vi "NI 9226 Getting Started (Host).vi"() -> ()   [LabVIEW 2018]
doc: "This VI will initialize the FPGA VI and then continually read and scale to temperature single point values from 4 channels of an analog input module."
uses:
  <vilib>/userdefined/High Color/nirio_resource_hc.ctl
  <vilib>/FPGAPlugInAG/cRIO-9045/niLvFpga_Open_cRIO-9045.vi
  <vilib>/rvi/interface/common/dynamic/niFpgaDynamicAddResources.vi
  <vilib>/FPGAPlugInAG/Dynamic/niLvFpga_Reset_Dynamic.vi
  <vilib>/Utility/error.llb/Error Cluster From Error Code.vi
  <vilib>/rvi/errors/niLvFpgaAdjustHostInterfaceError.vi
  <vilib>/FPGAPlugInAG/Dynamic/niLvFpga_Run_Dynamic.vi
  <vilib>/RVI Host/nirviSupport.llb/nirviErrorClusterFromErrorCode.vi
  <vilib>/FPGAPlugInAG/Dynamic/niLvFpga_Close_Dynamic.vi
  <vilib>/rvi/interface/nirviOpenFPGA/nirviOpenFPGA.xnode
  FPGA Bitfiles/crio_FPGATarget2_NI9226GettingSta_IIeFYHumF2U.lvbitx
  NI 9226 Getting Started (FPGA).vi
  <vilib>/rvi/interface/nirviMethod/nirviMethod.xnode
  <vilib>/rvi/interface/nirviReadWriteControl/nirviReadWriteControl.xnode
  <vilib>/rvi/interface/nirviCloseFPGA/nirviCloseFPGA.xnode
  <vilib>/rvi/interface/Simulation/niFpgaSimulationCallBeginRW.vi
  <vilib>/rvi/interface/nirviMethod/StockFPGA_InlinedMethodWaitForSingleIRQ.vi
  <vilib>/FPGAPlugInAG/Dynamic/niLvFpga_WaitOnIrq_Dynamic.vi
  <vilib>/FPGAPlugInAG/Dynamic/niLvFpga_AcknowledgeIrq_Dynamic.vi
  NiFpgaLv.dll
panel:
  in  "A":dbl=0.003908019978553057 format="%0.5e"
  in  "B":dbl=-5.774199962615967e-07
  in  "C":dbl=-4.182999866625403e-12 format="%0.5e"
  in  "Update":bool
  out "FPGA data transfer timed out":bool
  out "FPGA error out":errorcluster
  out "Host error out":errorcluster
  in  "Conversion Time":enum8{"200 ms", "2.5 ms"}(ring)
  in  "Resource name":T1="RIO0" caption="RIO Device"
  out "Coeff Out of Range":bool
  out "RTD Temperature":T2(graph)
  in  "stop":bool
  # "Overview: This example downloads and runs an FPGA VI that continuously reads single point values from 4 out of the 8 channel of the NI 9226\nRequirements: LabVIEW FPGA Module, LabVIEW Real-Time Module, NI-RIO\nInstructions: \n1) Modify timing parameters if desired . The timming parameters may also be changed during run-time using the \"Update\" button.\n2) Run the VI"
  # "Resource Parameters"
  # "Timing Parameters"
  # "RTD Parameters"
  # "Callendar-Van Dusen Constants"
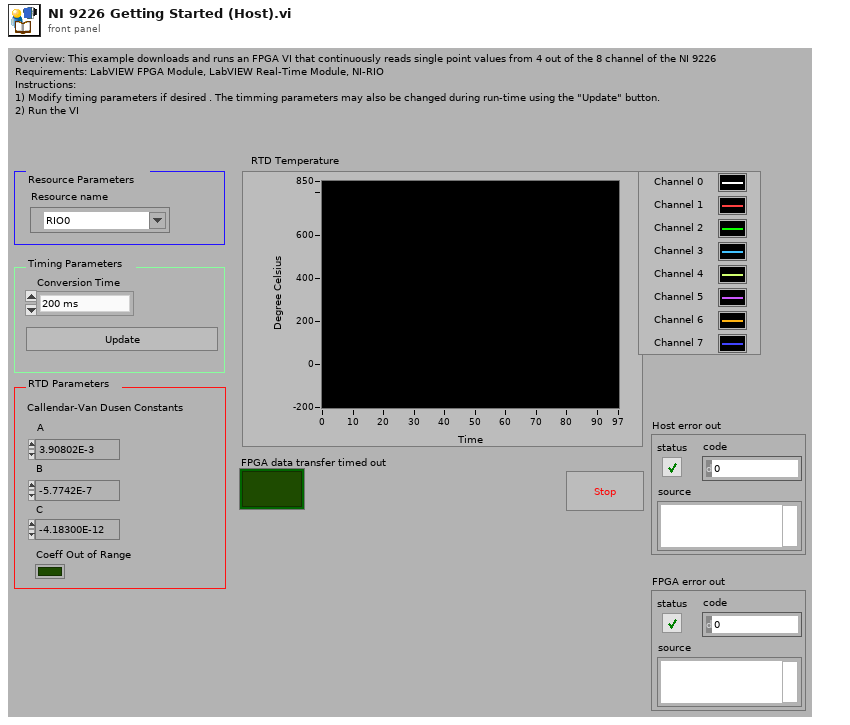
[diagram p1: front panel]
types:
  T1 = typedef "nirio_resource_hc.ctl" = tag
  T2 = cluster{"[0]":dbl, "[1]":dbl, "[2]":dbl, "[3]":dbl}
  T3 = cluster{"Mod6/RTD0":fxp<+/-,24,14>, "Mod6/RTD1":fxp<+/-,24,14>, "Mod6/RTD2":fxp<+/-,24,14>, "Mod6/RTD3":fxp<+/-,24,14>, "Mod6/RTD4":fxp<+/-,24,14>, "Mod6/RTD5":fxp<+/-,24,14>, "Mod6/RTD6":fxp<+/-,24,14>, "Mod6/RTD7":fxp<+/-,24,14>}
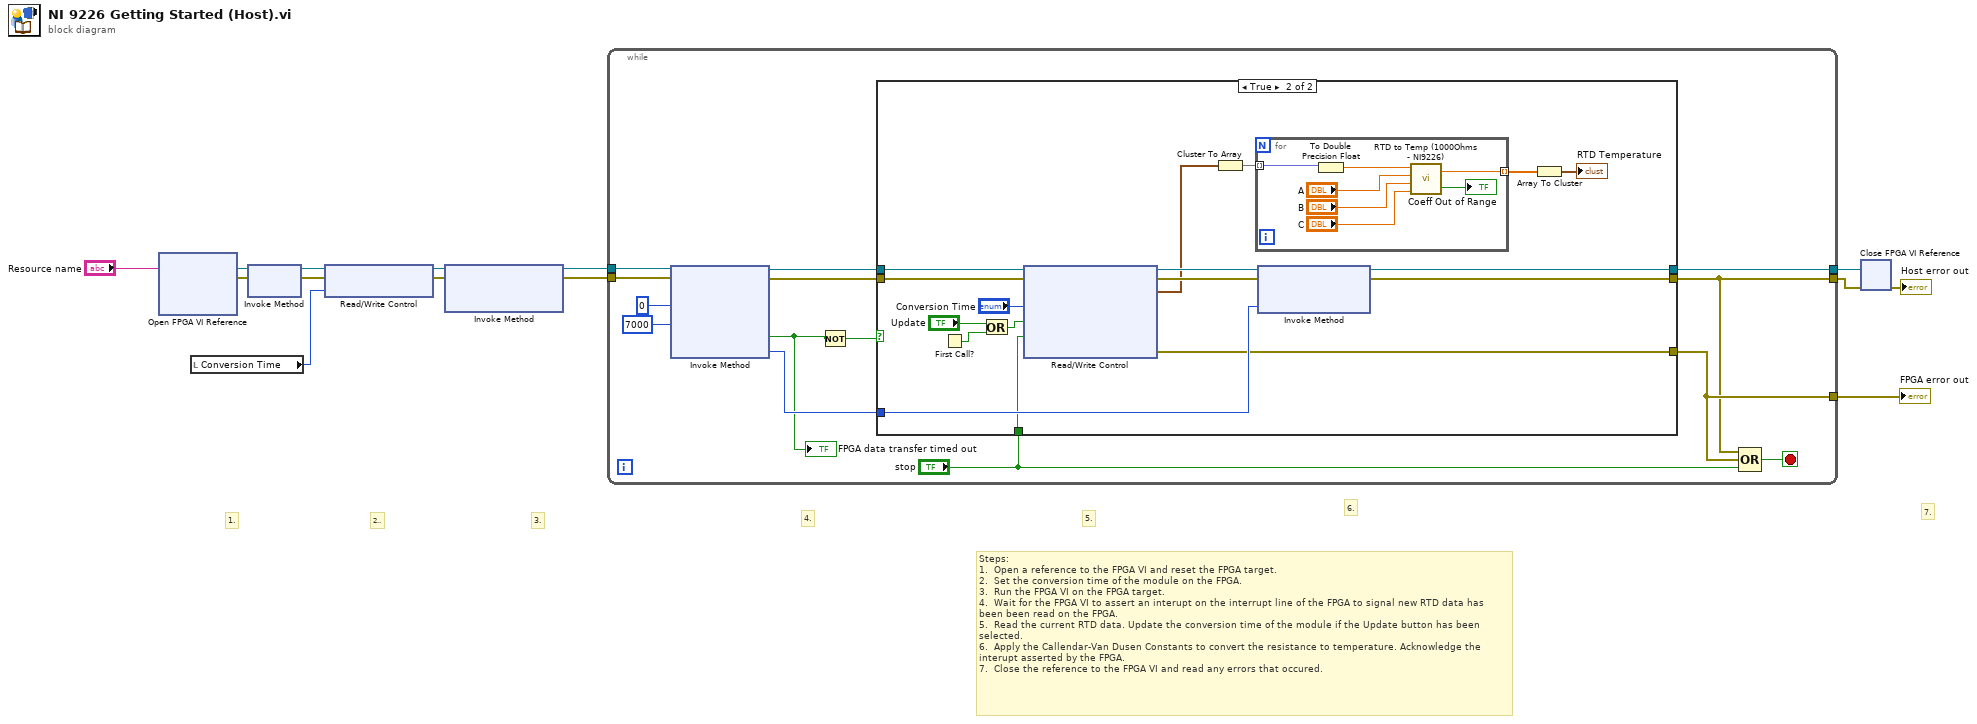
[diagram p0: block diagram]
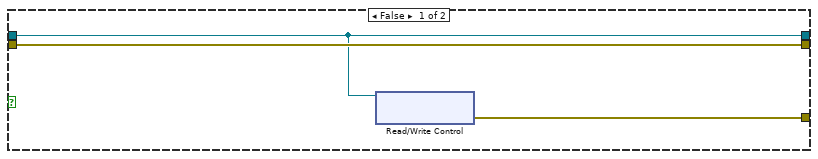
[diagram p2: hidden frame]
diagram:
  # "7."
  # "6."
  # "5."
  # "4."
  # "3."
  # "2.."
  # "1."
  # "Steps: \n1.  Open a reference to the FPGA VI and reset the FPGA target.\n2.  Set the conversion time of the module on the FPGA.\n3.  Run the FPGA VI on the FPGA target.\n4.  Wait for the FPGA VI to assert an interupt on the interrupt line of the FPGA to signal new RTD data has been been read on the FPGA.\n5.  Read the current RTD data. Update the conversion time of the module if the Update button has been selected.\n6.  Apply the Callendar-Van Dusen Constants to convert the resistance to temperature. Acknowledge the interupt asserted by the FPGA. \n7.  Close the reference to the FPGA VI and read any errors that occured."
  n1 = xnode "Open FPGA VI Reference"("resource name"="Resource name") -> ("FPGA VI Reference Out"=w2:refnum<k20>, "error out"=w1:errorcluster)  [unwired: 1 in]
  n2 = local read "Conversion Time"() -> (w5:enum8{"200 ms", "2.5 ms"})
  n3 = xnode "Invoke Method"("FPGA VI Reference In"=w2, "error in"=w1) -> ("FPGA VI Reference Out"=w4:refnum<k20>, "error out"=w3:errorcluster)
  n4 = xnode "Read/Write Control"("FPGA VI Reference In"=w4, "error in"=w3, "Conversion Time"=w5) -> ("FPGA VI Reference Out"=w13:refnum<k20>, "error out"=w14:errorcluster)
  n5 = xnode "Invoke Method"("FPGA VI Reference In"=w13, "error in"=w14) -> ("FPGA VI Reference Out"=w10:refnum<k20>, "error out"=w9:errorcluster)  [unwired: 1 in]
  n6 = while {
    tunnel: [w24] -> w12
    tunnel: [w15] -> w11
    tunnel: w10 -> [w21]
    tunnel: w9 -> [w20]
    tunnel: [w16] -> w6
    stop <- w22 stop-if-true
    n7 = xnode "Invoke Method"("FPGA VI Reference In"=w21, "error in"=w20, "IRQ Number(s)"=0, "Timeout (ms)"=7000 ("timeout (ms)(-1 for no timeout)")) -> ("FPGA VI Reference Out"=w26:refnum<k20>, "error out"=w25:errorcluster, "Timed Out"=w17:bool, "IRQ(s) Asserted"=w23:i32)
    "FPGA data transfer timed out" <- w17
    n8 = Not(x=w17) -> (.not. x?=w18:bool)
    n9 = case shown="True" w18 {
      tunnel: w26 -> [w30 w48]
      tunnel: w25 -> [w31 w47]
      tunnel: [w30 w45] -> w24
      tunnel: w23 -> [_ w44]
      tunnel: [w31 w43] -> w15
      tunnel: "stop" -> [_ w34]
      tunnel: [w29 w33] -> w16
      frame False {
        n10 = xnode "Read/Write Control"("FPGA VI Reference In"=w30) -> ("FPGA Error Out"=w29:errorcluster)  [unwired: 1 in, 2 out]
      }
      frame True {
        n11 = First Call?() -> (First Call?: T/F=w38:bool)
        n12 = Or(x="Update", y=w38) -> (x .or. y?=w32:bool)
        n13 = xnode "Read/Write Control"("FPGA VI Reference In"=w48, "error in"=w47, "Conversion Time"="Conversion Time", "Update Configuration"=w32, "stop"=w34) -> ("FPGA VI Reference Out"=w46:refnum<k20>, "error out"=w40:errorcluster, "RTD 9226 Ohms"=w35:T3, "FPGA Error Out"=w33:errorcluster)
        n14 = Cluster To Array(cluster=w35) -> (array=w42:fxp<+/-,24,14>[])
        n15 = for {
          tunnel: w42 -> [w53] mode=indexing
          tunnel: [w55] -> w41 mode=indexing
          n16 = To Double Precision Float(number=w53) -> (double precision float=w52:dbl)
          n17 = call "RTD to Temp (1000Ohms - NI9226).vi"("C"="C", "B"="B", "A"="A", "RTD Resistance"=w52) -> ("Coeff Out of Range"=→"Coeff Out of Range":bool, "RTDtemp"=w55:dbl)
        }
        n18 = xnode "Invoke Method"("FPGA VI Reference In"=w46, "error in"=w40, "IRQ Number(s)"=w44) -> ("FPGA VI Reference Out"=w45:refnum<k20>, "error out"=w43:errorcluster)
        n19 = Array To Cluster(array=w41) -> (cluster=→"RTD Temperature":T2)
      }
    }
    n20 = Compound Arithmetic op=OR(w15, w16, "stop") -> (w22:bool)
  }
  "FPGA error out" <- w6
  n21 = xnode "Close FPGA VI Reference"("FPGA VI Reference In"=w12, "error in"=w11) -> ("error out"=→"Host error out":errorcluster)
